vi "Export_Data_From_Excel_v1.3_Graph_XY_v1.0.vi"() -> ()   [LabVIEW 2018]
panel:
  out "XY Graph":cluster{dbl[], dbl[]}(graph)
  out "Array 2":dbl[][](array[numeric])
  in  "Open":bool
  in  "Загрузка Excel приложения":refnum<k7>
  in  "Excel._Worksheet 2":refnum<k7>
  in  "Array":string[][](array[string])
  in  "Выбор файла":path
  # "Y"
  # "Z"
  # "№ отм."
  # "X"
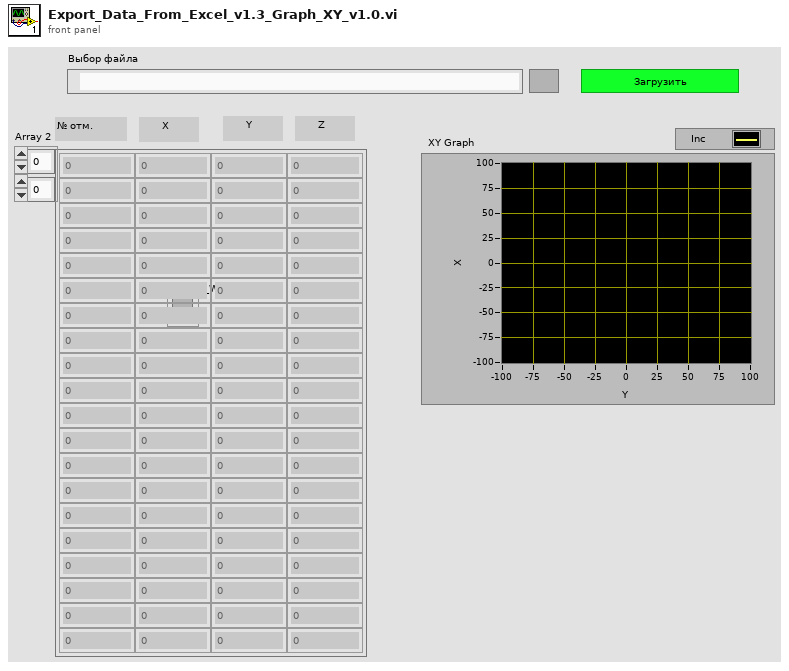
[diagram p1: front panel]
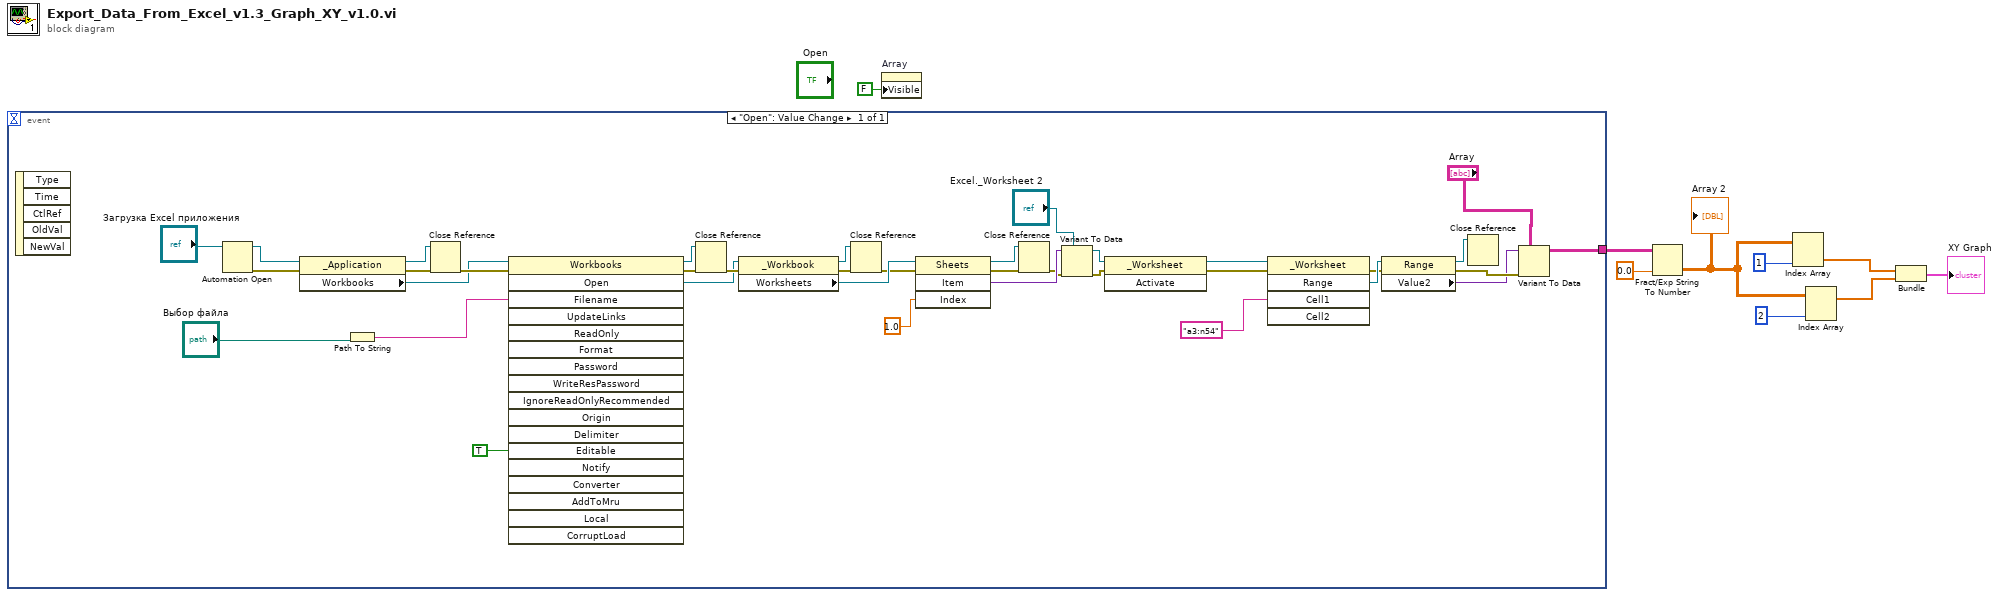
[diagram p0: block diagram]
diagram:
  n1 = event shown="[0] \"Open\": Value Change" {
    selector: _ -> [_]
    dyn-events: _ -> [_]
    timeout: _ -> [_]
    tunnel: [w13] -> w7
    event "Open": Value Change {
      n2 = event-data() -> ()  [unwired: 1 in, 5 out]
      n3 = Automation Open(Automation Refnum="Загрузка Excel приложения") -> (Automation Refnum=w45:refnum<k7>, error out=w33:errorcluster)  [unwired: 3 in]
      n4 = property class="_Application"(reference=w45, error in=w33) -> (reference out=w31:refnum<k7>, error out=w26:errorcluster, "Workbooks"=w16:refnum<k7>)
      n5 = Path To String(path="Выбор файла") -> (string=w14:string)
      n6 = Close Reference(reference=w31, error in (no error)=w26) -> (error out=w25:errorcluster)
      n7 = invoke class="Workbooks" method="Open"(reference=w16, error in=w25, "Filename"=w14, "Editable"=TRUE) -> (reference out=w30:refnum<k7>, error out=w24:errorcluster, "Open"=w15:refnum<k7>)  [unwired: 14 in, 15 out]
      n8 = Close Reference(reference=w30, error in (no error)=w24) -> (error out=w23:errorcluster)
      n9 = property class="_Workbook"(reference=w15, error in=w23) -> (reference out=w29:refnum<k7>, error out=w22:errorcluster, "Worksheets"=w40:refnum<k7>)
      n10 = Close Reference(reference=w29, error in (no error)=w22) -> (error out=w21:errorcluster)
      n11 = invoke class="Sheets" method="Item"(reference=w40, error in=w21, "Index"=1.0) -> (reference out=w28:refnum<k7>, error out=w20:errorcluster, "Item"=w41:variant)  [unwired: 1 in, 1 out]
      n12 = Close Reference(reference=w28, error in (no error)=w20) -> (error out=w19:errorcluster)
      n13 = Variant To Data(error in=w19, type="Excel._Worksheet 2", Variant=w41) -> (data=w43:refnum<k7>, error out=w32:errorcluster)
      n14 = invoke class="_Worksheet" method="Activate"(reference=w43, error in=w32) -> (reference out=w34:refnum<k7>, error out=w18:errorcluster)  [unwired: 1 in, 1 out]
      n15 = invoke class="_Worksheet" method="Range"(reference=w34, error in=w18, "Cell1"="a3:n54") -> (error out=w17:errorcluster, "Range"=w36:refnum<k7>)  [unwired: 2 in, 3 out]
      n16 = property class="Range"(reference=w36, error in=w17) -> (reference out=w27:refnum<k7>, error out=w38:errorcluster, "Value2"=w37:variant)
      n17 = Close Reference(reference=w27) -> ()  [unwired: 1 in, 1 out]
      n18 = Variant To Data(error in=w38, type="Array", Variant=w37) -> (data=w13:string[][])  [unwired: 1 out]
    }
  }
  n19 = property on="Array" class="Arr (strict)"("Visible"=FALSE) -> ()  [unwired: 2 in, 2 out]
  n20 = Fract/Exp String To Number(string=w7, default (0 dbl)=0.0) -> (number=w4:dbl[][])  [unwired: 2 in, 1 out]
  "Array 2" <- w4
  n21 = Index Array(array=w4, index (col)=1) -> (element=w2:dbl[])  [unwired: 1 in]
  n22 = Index Array(array=w4, index (col)=2) -> (element=w3:dbl[])  [unwired: 1 in]
  n23 = Bundle(w2, w3) -> (→"XY Graph":cluster{dbl[], dbl[]})  [unwired: 1 in]
